vi "双路双通通断器（DBL）.vi"(7 "默认值":dbl=nan, 9 "直通？":bool=TRUE, 10 "Y_In":dbl, 11 "X_In":dbl) -> (2 "Y_Out":dbl, 3 "X_Out":dbl)   [LabVIEW 2012]
doc: "功能：\n\n返回一个枚举，表明输入数的范围，用于三段比较。\n\n\nCSXCS_366创建。"
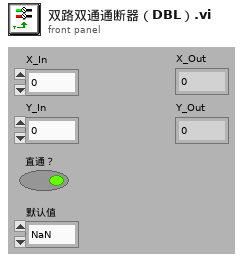
[diagram p1: front panel]
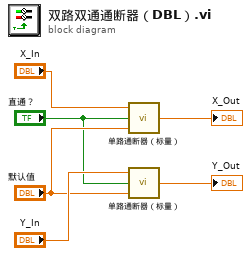
[diagram p0: block diagram]
diagram:
  n1 = call-poly "单路通断器（标量）.vi"("默认值"="默认值", "直通？"="直通？", "X_In"="X_In") -> ("X_Out"=→"X_Out":dbl)
  n2 = call-poly "单路通断器（标量）.vi"("默认值"="默认值", "直通？"="直通？", "X_In"="Y_In") -> ("X_Out"=→"Y_Out":dbl)
